vi "Wavelength_Tables_NeHgAr.vi"() -> ()   [LabVIEW 2021]
panel:
  out "Standard Wavelengths":cluster{"Y":dbl[], "Y":dbl[]}[](graph)=[{"Y"=[302.70159912109375, 302.88641357421875, 319.8586120605469, 332.37451171875, 337.82159423828125, 352.047119140625, 376.6258850097656, 377.7132873535156, 540.05615234375, 585.248779296875, 602.9996948242188, 607.4337768554688, 614.3062744140625, 616.359375, 621.7281494140625, 626.6494750976562, 638.2991943359375, 640.2247924804688, 650.65283203125, 659.895263671875, 692.9467163085938, 703.2413330078125, 717.393798828125, 724.5166625976562, 837.7608032226562, 865.4382934570312, 878.062255859375, 878.3753051757812, 1114.302001953125, 1117.75244140625, 1152.2745361328125], "Y"=[300.0, 300.0, 500.0, 1000.0, 500.0, 100.0, 800.0, 1000.0, 200.0, 200.0, 100.0, 100.0, 100.0, 100.0, 100.0, 100.0, 100.0, 200.0, 150.0, 100.0, 1000.0, 800.0, 800.0, 800.0, 800.0, 600.0, 600.0, 400.0, 300.0, 500.0, 300.0]}, {"Y"=[205.28280639648438, 226.22230529785156, 253.65170288085938, 284.7674865722656, 296.7279968261719, 365.0152893066406, 398.3930969238281, 404.65631103515625, 435.8327941894531, 542.5253295898438, 546.073486328125, 567.7105102539062, 614.947509765625, 794.4555053710938, 1013.9760131835938], "Y"=[400.0, 400.0, 1000.0, 400.0, 250.0, 600.0, 1000.0, 400.0, 1000.0, 80.0, 500.0, 200.0, 250.0, 250.0, 200.0]}, {"Y"=[427.7528076171875, 434.806396484375, 460.9566955566406, 472.6867980957031, 476.48651123046875, 480.60198974609375, 487.98638916015625, 696.5430908203125, 706.7218017578125, 750.3869018554688, 763.5106201171875, 794.817626953125, 800.61572265625, 801.4785766601562, 810.3693237304688, 811.5311279296875, 912.2966918945312, 965.7786254882812], "Y"=[200.0, 250.0, 200.0, 200.0, 250.0, 200.0, 250.0, 300.0, 300.0, 600.0, 700.0, 600.0, 600.0, 700.0, 600.0, 1000.0, 1000.0, 700.0]}]
  in  "Int_Ne":dbl[](array[numeric])=[300.0, 300.0, 500.0, 1000.0, 500.0, 100.0, 800.0, 1000.0, 200.0, 200.0, 100.0, 100.0, 100.0, 100.0, 100.0, 100.0, 100.0, 200.0, 150.0, 100.0, 1000.0, 800.0, 800.0, 800.0, 800.0, 600.0, 600.0, 400.0, 300.0, 500.0, 300.0]
  in  "WL_Ne":dbl[](array[numeric])=[302.70159912109375, 302.88641357421875, 319.8586120605469, 332.37451171875, 337.82159423828125, 352.047119140625, 376.6258850097656, 377.7132873535156, 540.05615234375, 585.248779296875, 602.9996948242188, 607.4337768554688, 614.3062744140625, 616.359375, 621.7281494140625, 626.6494750976562, 638.2991943359375, 640.2247924804688, 650.65283203125, 659.895263671875, 692.9467163085938, 703.2413330078125, 717.393798828125, 724.5166625976562, 837.7608032226562, 865.4382934570312, 878.062255859375, 878.3753051757812, 1114.302001953125, 1117.75244140625, 1152.2745361328125] format="%#_8g"
  in  "Int_Hg":dbl[](array[numeric])=[400.0, 400.0, 1000.0, 400.0, 250.0, 600.0, 1000.0, 400.0, 1000.0, 80.0, 500.0, 200.0, 250.0, 250.0, 200.0]
  in  "WL_Hg":dbl[](array[numeric])=[205.28280639648438, 226.22230529785156, 253.65170288085938, 284.7674865722656, 296.7279968261719, 365.0152893066406, 398.3930969238281, 404.65631103515625, 435.8327941894531, 542.5253295898438, 546.073486328125, 567.7105102539062, 614.947509765625, 794.4555053710938, 1013.9760131835938] format="%#_8g"
  in  "Int_Ar":dbl[](array[numeric])=[200.0, 250.0, 200.0, 200.0, 250.0, 200.0, 250.0, 300.0, 300.0, 600.0, 700.0, 600.0, 600.0, 700.0, 600.0, 1000.0, 1000.0, 700.0]
  in  "WL_Ar":dbl[](array[numeric])=[427.7528076171875, 434.806396484375, 460.9566955566406, 472.6867980957031, 476.48651123046875, 480.60198974609375, 487.98638916015625, 696.5430908203125, 706.7218017578125, 750.3869018554688, 763.5106201171875, 794.817626953125, 800.61572265625, 801.4785766601562, 810.3693237304688, 811.5311279296875, 912.2966918945312, 965.7786254882812] format="%#_8g"
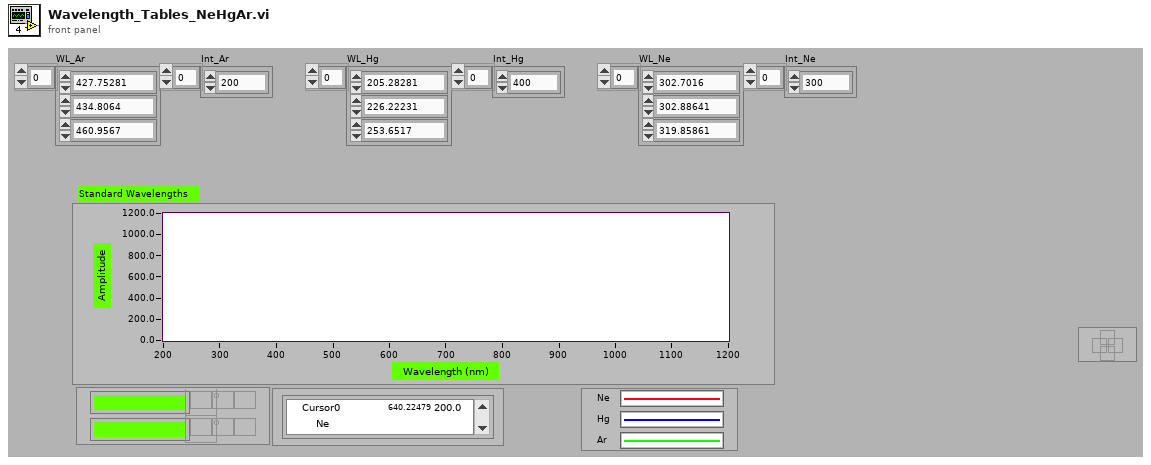
[diagram p1: front panel]
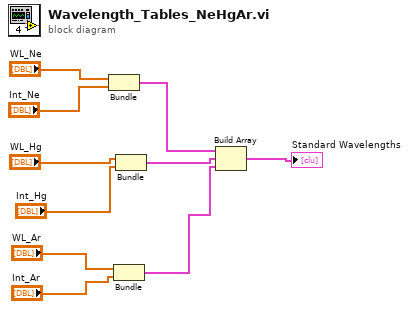
[diagram p0: block diagram]
diagram:
  n1 = Bundle("WL_Ne"="WL_Ne", "Int_Ne"="Int_Ne") -> (w4:cluster{"WL_Ne":dbl[], "Int_Ne":dbl[]})  [unwired: 1 in]
  n2 = Bundle("WL_Ar"="WL_Ar", "Int_Ar"="Int_Ar") -> (w2:cluster{"WL_Ar":dbl[], "Int_Ar":dbl[]})  [unwired: 1 in]
  n3 = Bundle("WL_Hg"="WL_Hg", "Int_Hg"="Int_Hg") -> (w3:cluster{"WL_Hg":dbl[], "Int_Hg":dbl[]})  [unwired: 1 in]
  n4 = Build Array(w4, w3, w2) -> (→"Standard Wavelengths":cluster{"WL_Ar":dbl[], "Int_Ar":dbl[]}[])
